vi "Set Server Address.vi"(10 "Server Address":string, 11 "OOP Server in":refnum<class "Query Server.lvclass">) -> (3 "OOP Server out":refnum<class "Query Server.lvclass">)   [LabVIEW 2019, in "Query Server.lvlib" / "Query Server.lvclass"]
uses:
  Query Server.lvclass
  Query Server.lvclass/Query Server.ctl
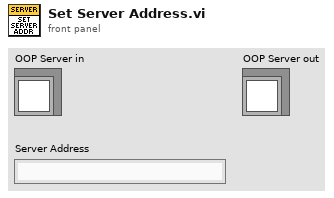
[diagram p1: front panel]
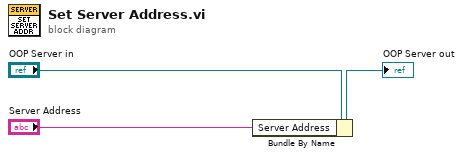
[diagram p0: block diagram]
diagram:
  n1 = Bundle By Name(cluster="OOP Server in", "Server Address"="Server Address") -> (→"OOP Server out":refnum<class "Query Server.lvclass">)
